vi "addFIFO.vi"(8 "error in (no error)":errorcluster, 10 "Frame":T1 {"Data" format="%02x"}, 11 "Mockbus in":refnum<class "Mockbus.lvclass">) -> (0 "error out":errorcluster, 3 "Mockbus out":refnum<class "Mockbus.lvclass">)   [LabVIEW 2015, in "Mockbus.lvclass"]
uses:
  Mockbus.lvclass
  Typedefs/Frame.ctl
  Mockbus.lvclass/Mockbus.ctl
  Typedefs/RTTypeDefs.lvlib
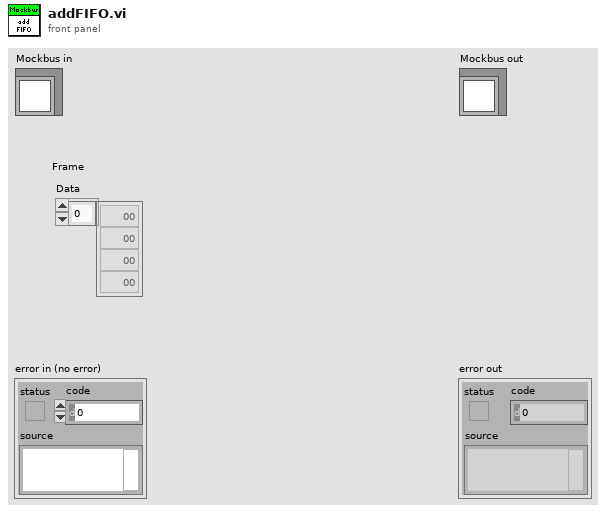
[diagram p1: front panel]
types:
  T1 = typedef "RTTypeDefs.lvlib/Frame.ctl" = cluster{"Data":u8[]}
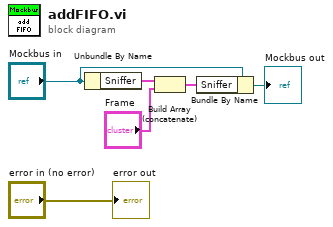
[diagram p0: block diagram]
diagram:
  n1 = Unbundle By Name("Mockbus in") -> ("Sniffer"=w5:T1[])
  n2 = Build Array (concatenate)(w5, "Frame") -> (w3:T1[])
  n3 = Bundle By Name(cluster="Mockbus in", "Sniffer"=w3) -> (→"Mockbus out":refnum<class "Mockbus.lvclass">)
  "error out" <- "error in (no error)"
